vi "SendTDT8.vi"(1 "String":string, 4 "Mode":T1(ring)) -> ()   [LabVIEW 2013]
uses:
  <vilib>/DAQmx/write.llb/DAQmx Write (Digital 1D Bool 1Chan 1Samp).vi
  <vilib>/DAQmx/miscellaneous.llb/DAQmx Fill In Error Info.vi
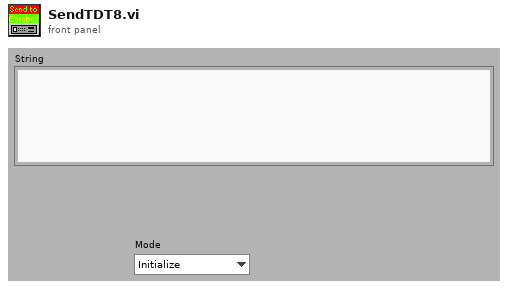
[diagram p1: front panel]
types:
  T1 = enum16{"Initialize", "String", "Start", "New Session", "Stop", "Resume", "Close"}
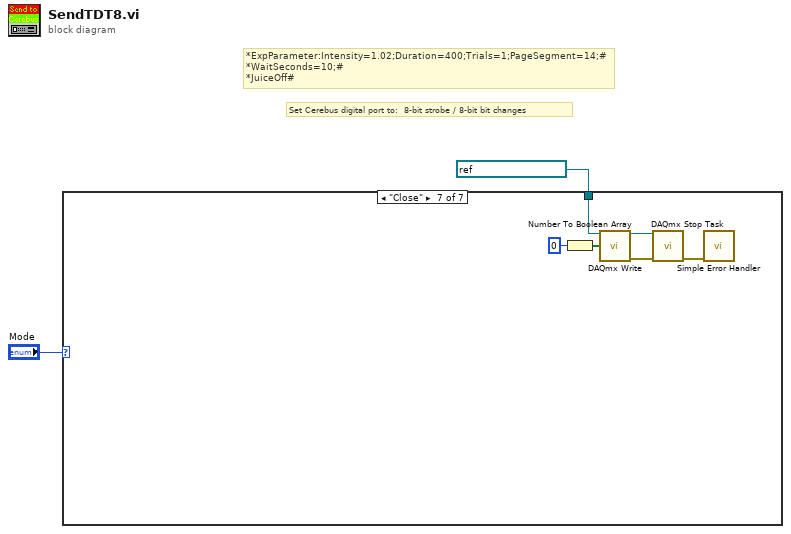
[diagram p0: block diagram]
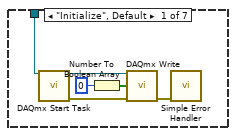
[diagram p2: hidden frame]
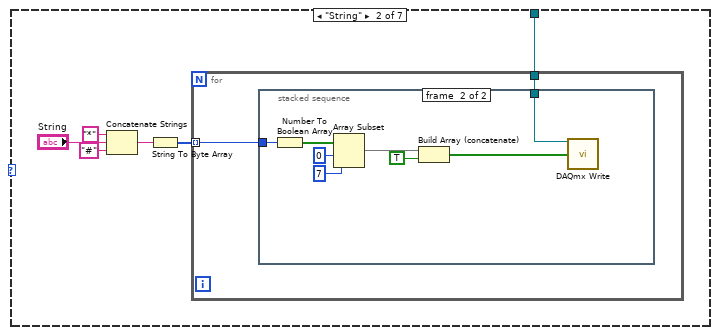
[diagram p3: hidden frame]
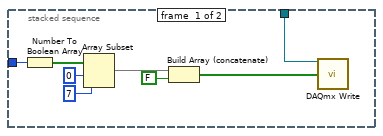
[diagram p4: hidden frame]
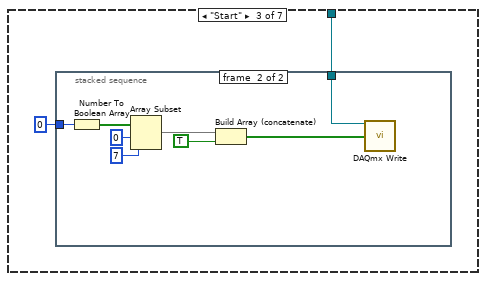
[diagram p5: hidden frame]
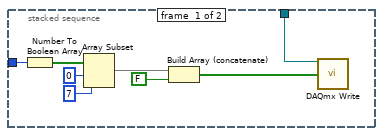
[diagram p6: hidden frame]
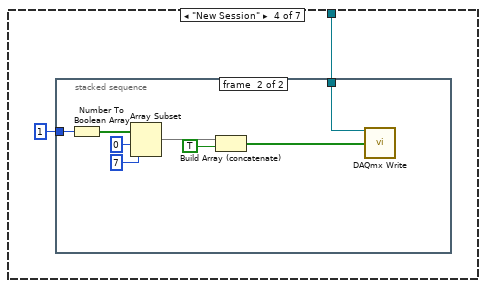
[diagram p7: hidden frame]
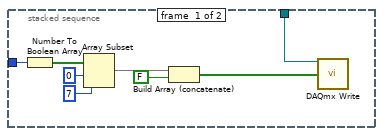
[diagram p8: hidden frame]
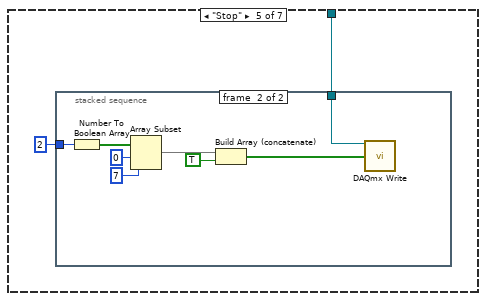
[diagram p9: hidden frame]
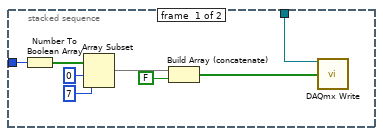
[diagram p10: hidden frame]
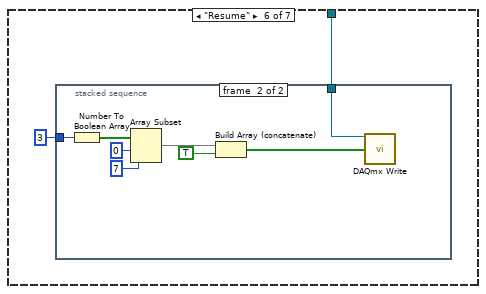
[diagram p11: hidden frame]
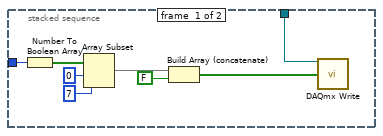
[diagram p12: hidden frame]
diagram:
  # "Set Cerebus digital port to:  8-bit strobe / 8-bit bit changes"
  # "*ExpParameter:Intensity=1.02;Duration=400;Trials=1;PageSegment=14;#\n*WaitSeconds=10;#\n*JuiceOff#"
  n1 = case shown="\"Close\"" "Mode" {
    tunnel: refnum<k21> "cerebus_markers" ("task/channels in") -> [w8 w9 w34 w52 w70 w88 w106]
    frame "Initialize", Default {
      n2 = call <vilib>:"DAQmx Start Task.vi"("task/channels in"=w8) -> ("task out"=w7:refnum<k21>, "error out"=w6:errorcluster)  [unwired: 13 in]
      n3 = Number To Boolean Array(number=u8 0) -> (Boolean array=w4:bool[])
      n4 = call-poly <vilib>:"DAQmx Write.vi"("task/channels in"=w7, "data"=w4, "error in"=w6) -> ("error out"=w3:errorcluster)  [unwired: 10 in, 2 out]
      n5 = call <vilib>:"Simple Error Handler.vi"("error in (no error)"=w3) -> ()  [unwired: 4 in, 5 out]
    }
    frame "String" {
      n6 = Concatenate Strings("*", "String", "#" ("string")) -> (w11:string)
      n7 = String To Byte Array(string=w11) -> (unsigned byte array=w14:u8[])
      n8 = for {
        tunnel: w14 -> [w15] mode=indexing
        tunnel: w9 -> [w16]
        n9 = stacked-sequence {
          tunnel: w15 -> [w24 w27]
          tunnel: w16 -> [w23 w32]
          frame #0 {
            n10 = Number To Boolean Array(number=w24) -> (Boolean array=w22:bool[])
            n11 = Array Subset(array=w22, index=0, length=7) -> (w19:bool[])
            n12 = Build Array (concatenate)(w19, FALSE) -> (w18:bool[])
            n13 = call-poly <vilib>:"DAQmx Write.vi"("task/channels in"=w23, "data"=w18) -> ()  [unwired: 11 in, 3 out]
          }
          frame #1 {
            n14 = Number To Boolean Array(number=w27) -> (Boolean array=w31:bool[])
            n15 = Array Subset(array=w31, index=0, length=7) -> (w28:bool[])
            n16 = Build Array (concatenate)(w28, TRUE) -> (w26:bool[])
            n17 = call-poly <vilib>:"DAQmx Write.vi"("task/channels in"=w32, "data"=w26) -> ()  [unwired: 11 in, 3 out]
          }
        }
      }
    }
    frame "Start" {
      n18 = stacked-sequence {
        tunnel: u8 0 -> [w42 w45]
        tunnel: w34 -> [w41 w50]
        frame #0 {
          n19 = Number To Boolean Array(number=w42) -> (Boolean array=w40:bool[])
          n20 = Array Subset(array=w40, index=0, length=7) -> (w37:bool[])
          n21 = Build Array (concatenate)(w37, FALSE) -> (w36:bool[])
          n22 = call-poly <vilib>:"DAQmx Write.vi"("task/channels in"=w41, "data"=w36) -> ()  [unwired: 11 in, 3 out]
        }
        frame #1 {
          n23 = Number To Boolean Array(number=w45) -> (Boolean array=w49:bool[])
          n24 = Array Subset(array=w49, index=0, length=7) -> (w46:bool[])
          n25 = Build Array (concatenate)(w46, TRUE) -> (w44:bool[])
          n26 = call-poly <vilib>:"DAQmx Write.vi"("task/channels in"=w50, "data"=w44) -> ()  [unwired: 11 in, 3 out]
        }
      }
    }
    frame "New Session" {
      n27 = stacked-sequence {
        tunnel: u8 1 -> [w60 w63]
        tunnel: w52 -> [w59 w68]
        frame #0 {
          n28 = Number To Boolean Array(number=w60) -> (Boolean array=w58:bool[])
          n29 = Array Subset(array=w58, index=0, length=7) -> (w55:bool[])
          n30 = Build Array (concatenate)(w55, FALSE) -> (w54:bool[])
          n31 = call-poly <vilib>:"DAQmx Write.vi"("task/channels in"=w59, "data"=w54) -> ()  [unwired: 11 in, 3 out]
        }
        frame #1 {
          n32 = Number To Boolean Array(number=w63) -> (Boolean array=w67:bool[])
          n33 = Array Subset(array=w67, index=0, length=7) -> (w64:bool[])
          n34 = Build Array (concatenate)(w64, TRUE) -> (w62:bool[])
          n35 = call-poly <vilib>:"DAQmx Write.vi"("task/channels in"=w68, "data"=w62) -> ()  [unwired: 11 in, 3 out]
        }
      }
    }
    frame "Stop" {
      n36 = stacked-sequence {
        tunnel: u8 2 -> [w78 w81]
        tunnel: w70 -> [w77 w86]
        frame #0 {
          n37 = Number To Boolean Array(number=w78) -> (Boolean array=w76:bool[])
          n38 = Array Subset(array=w76, index=0, length=7) -> (w73:bool[])
          n39 = Build Array (concatenate)(w73, FALSE) -> (w72:bool[])
          n40 = call-poly <vilib>:"DAQmx Write.vi"("task/channels in"=w77, "data"=w72) -> ()  [unwired: 11 in, 3 out]
        }
        frame #1 {
          n41 = Number To Boolean Array(number=w81) -> (Boolean array=w85:bool[])
          n42 = Array Subset(array=w85, index=0, length=7) -> (w82:bool[])
          n43 = Build Array (concatenate)(w82, TRUE) -> (w80:bool[])
          n44 = call-poly <vilib>:"DAQmx Write.vi"("task/channels in"=w86, "data"=w80) -> ()  [unwired: 11 in, 3 out]
        }
      }
    }
    frame "Resume" {
      n45 = stacked-sequence {
        tunnel: u8 3 -> [w96 w99]
        tunnel: w88 -> [w95 w104]
        frame #0 {
          n46 = Number To Boolean Array(number=w96) -> (Boolean array=w94:bool[])
          n47 = Array Subset(array=w94, index=0, length=7) -> (w91:bool[])
          n48 = Build Array (concatenate)(w91, FALSE) -> (w90:bool[])
          n49 = call-poly <vilib>:"DAQmx Write.vi"("task/channels in"=w95, "data"=w90) -> ()  [unwired: 11 in, 3 out]
        }
        frame #1 {
          n50 = Number To Boolean Array(number=w99) -> (Boolean array=w103:bool[])
          n51 = Array Subset(array=w103, index=0, length=7) -> (w100:bool[])
          n52 = Build Array (concatenate)(w100, TRUE) -> (w98:bool[])
          n53 = call-poly <vilib>:"DAQmx Write.vi"("task/channels in"=w104, "data"=w98) -> ()  [unwired: 11 in, 3 out]
        }
      }
    }
    frame "Close" {
      n54 = Number To Boolean Array(number=u8 0) -> (Boolean array=w109:bool[])
      n55 = call-poly <vilib>:"DAQmx Write.vi"("task/channels in"=w106, "data"=w109) -> ("task out"=w108:refnum<k21>, "error out"=w107:errorcluster)  [unwired: 11 in, 1 out]
      n56 = call <vilib>:"DAQmx Stop Task.vi"("task/channels in"=w108, "error in"=w107) -> ("error out"=w105:errorcluster)  [unwired: 12 in, 1 out]
      n57 = call <vilib>:"Simple Error Handler.vi"("error in (no error)"=w105) -> ()  [unwired: 4 in, 5 out]
    }
  }
